vi "MCCETC01_Main.vi"(7 "stop_external":refnum<vi>) -> ()   [LabVIEW 2019]
uses:
  MCCETC_Global.vi
panel:
  out "T7":dbl format="%.2f"
  in  "Logging":bool=TRUE
  out "status_log":bool caption="Status"
  out "T6":dbl format="%.2f"
  out "T5":dbl format="%.2f"
  out "T4":dbl format="%.2f"
  out "T3":dbl format="%.2f"
  out "T2":dbl format="%.2f"
  in  "Tab Control":enum32{"Top Coil", "Bottom Coil"}(tab)
  out "T0 Chart":waveform(dbl)[](graph)
  out "T1 Chart":waveform(dbl)[](graph)
  out "T2 Chart":waveform(dbl)[](graph)
  out "T3 Chart":waveform(dbl)[](graph)
  out "T4 Chart":waveform(dbl)[](graph)
  out "T5 Chart":waveform(dbl)[](graph)
  out "T6 Chart":waveform(dbl)[](graph)
  out "T7 Chart":waveform(dbl)[](graph)
  in  "Readout Interval":i32=5 caption="sec"
  in  "units":i32(ring)=2 items=["degC", "degF", "kelvin", "raw"]
  out "T1":dbl format="%.2f"
  out "T0":dbl format="%.2f"
  out "Readout Status":bool
  out "Last Measured":timestamp format="%<%Y-%m-%d %H:%M:%S>T"
  in  "stop":bool
  # "MCC E-TC #01:  Target Magnet Coil"
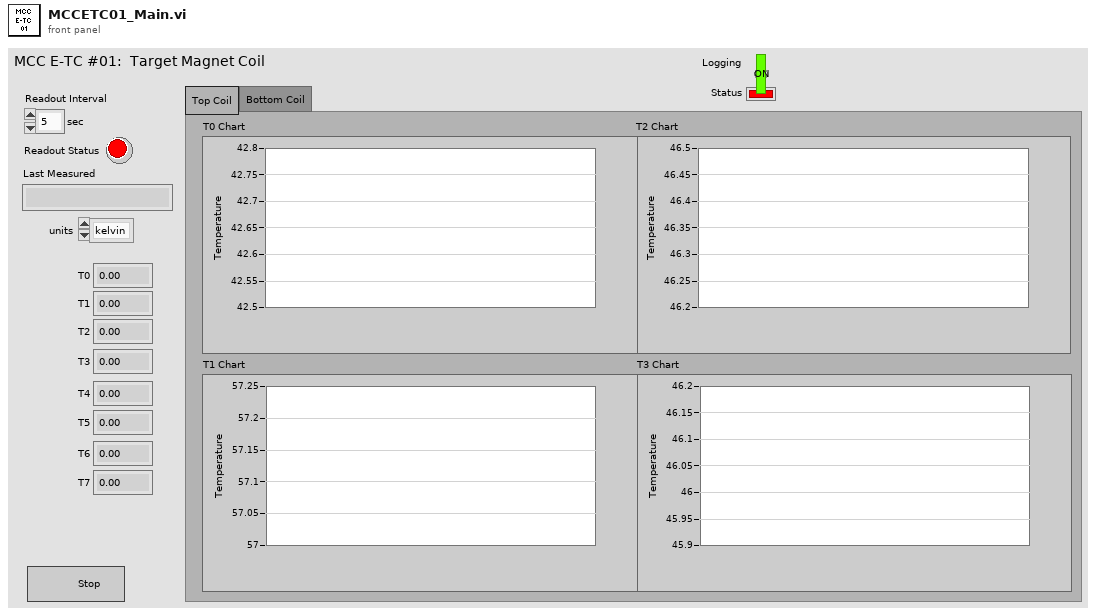
[diagram p1: front panel]
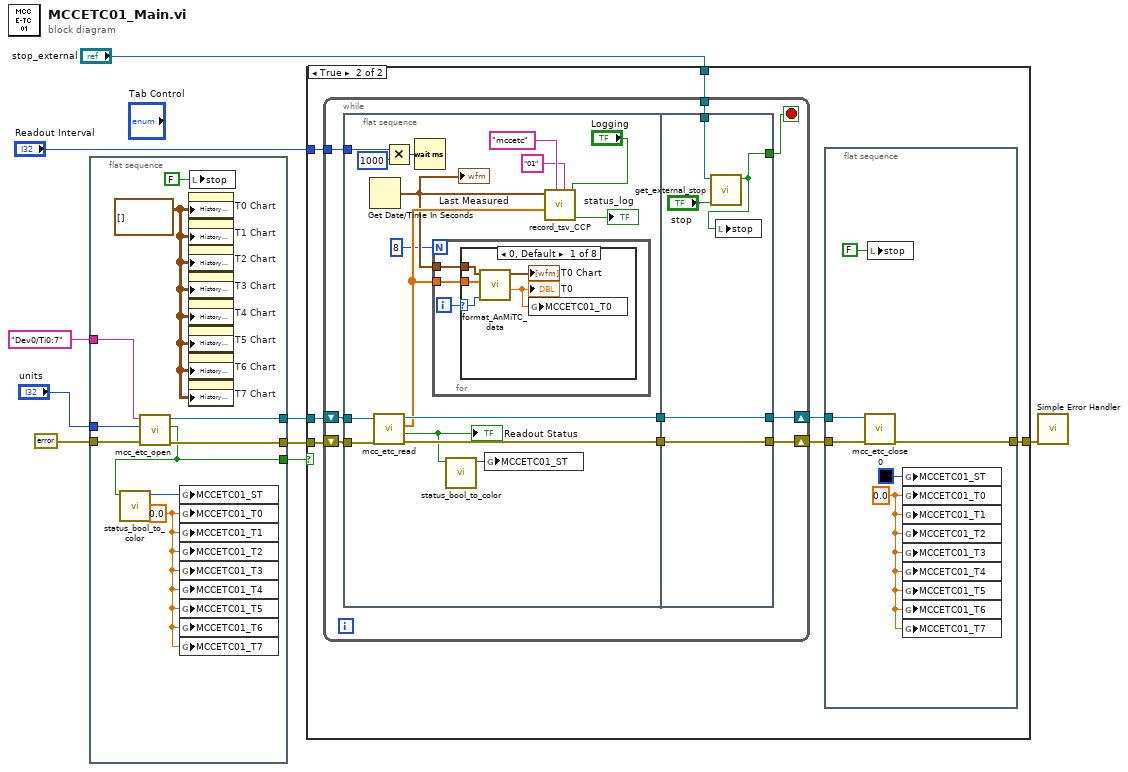
[diagram p0: block diagram]
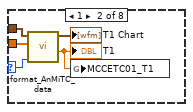
[diagram p3: hidden frame]
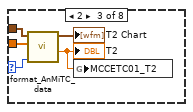
[diagram p4: hidden frame]
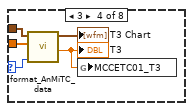
[diagram p5: hidden frame]
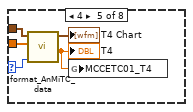
[diagram p6: hidden frame]
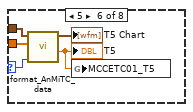
[diagram p7: hidden frame]
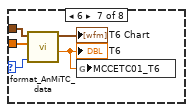
[diagram p8: hidden frame]
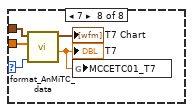
[diagram p9: hidden frame]
diagram:
  n1 = flat-sequence {
    tunnel: [w19] -> w9
    tunnel: errorcluster {"status"=FALSE, "code"=0, "source"=""} ("error in") -> [w18]
    tunnel: [w17] -> w7
    tunnel: "Dev0/Ti0:7" ("Device/Channel Name") -> [w16]
    tunnel: "units" -> [w15]
    tunnel: [w10] -> w2
    frame #0 {
      w12 = 0.0 ("MCCETC01_T0")
      w13 = waveform(dbl)[][] [] ("History Data")
      n2 = call "mcc_etc_open.vi"("error in"=w18, "units"=w15, "name"=w16) -> ("error out"=w17:errorcluster, "status"=w10:bool, "task out"=w19:refnum<k24>)  [unwired: 6 in]
      n3 = call "status_bool_to_color.vi"("status_bool_1"=w10) -> ("status_color"=w11:u32)  [unwired: 10 in]
      n4 = global write "MCCETC_Global.vi" "MCCETC01_ST"(w11) -> ()
      n5 = global write "MCCETC_Global.vi" "MCCETC01_T0"(w12) -> ()
      n6 = global write "MCCETC_Global.vi" "MCCETC01_T1"(w12) -> ()
      n7 = global write "MCCETC_Global.vi" "MCCETC01_T2"(w12) -> ()
      n8 = global write "MCCETC_Global.vi" "MCCETC01_T3"(w12) -> ()
      n9 = global write "MCCETC_Global.vi" "MCCETC01_T4"(w12) -> ()
      n10 = global write "MCCETC_Global.vi" "MCCETC01_T5"(w12) -> ()
      n11 = global write "MCCETC_Global.vi" "MCCETC01_T6"(w12) -> ()
      n12 = global write "MCCETC_Global.vi" "MCCETC01_T7"(w12) -> ()
      n13 = property on="T0 Chart" class="WFChart (strict)"("History Data"=w13) -> ()  [unwired: 2 in, 2 out]
      n14 = property on="T1 Chart" class="WFChart (strict)"("History Data"=w13) -> ()  [unwired: 2 in, 2 out]
      n15 = property on="T2 Chart" class="WFChart (strict)"("History Data"=w13) -> ()  [unwired: 2 in, 2 out]
      n16 = property on="T3 Chart" class="WFChart (strict)"("History Data"=w13) -> ()  [unwired: 2 in, 2 out]
      n17 = property on="T4 Chart" class="WFChart (strict)"("History Data"=w13) -> ()  [unwired: 2 in, 2 out]
      n18 = property on="T5 Chart" class="WFChart (strict)"("History Data"=w13) -> ()  [unwired: 2 in, 2 out]
      n19 = property on="T6 Chart" class="WFChart (strict)"("History Data"=w13) -> ()  [unwired: 2 in, 2 out]
      n20 = property on="T7 Chart" class="WFChart (strict)"("History Data"=w13) -> ()  [unwired: 2 in, 2 out]
      n21 = local write "stop"(FALSE ("Stop")) -> ()
    }
  }
  n22 = case shown="True" w2 {
    tunnel: w9 -> [_ w27]
    tunnel: w7 -> [w20 w26]
    tunnel: "Readout Interval" -> [_ w23]
    tunnel: [w20 w22] -> w3
    tunnel: "stop_external" -> [_ w21]
    frame False {
    }
    frame True {
      n23 = while {
        shift-right: [w40] -> w24
        shift-left: w26 -> [w41]
        shift-right: [w39] -> w25
        shift-left: w27 -> [w42]
        tunnel: w23 -> [w38]
        tunnel: w21 -> [w34]
        stop <- w35 stop-if-true
        n24 = flat-sequence {
          tunnel: w42 -> [w58]
          tunnel: w41 -> [w57]
          tunnel: w38 -> [w54]
          tunnel: [w56] -> w37
          tunnel: [w55] -> w36
          tunnel: [w105] -> w39
          tunnel: [w106] -> w40
          tunnel: w37 -> [w106]
          tunnel: w36 -> [w105]
          tunnel: [w103] -> w35
          tunnel: w34 -> [w102]
          frame #0 {
            n25 = Get Date/Time In Seconds() -> (seconds since 1Jan1904=w45:timestamp)
            "Last Measured" <- w45
            n26 = call "mcc_etc_read.vi"("error in"=w57, "task in"=w58) -> ("error out"=w56:errorcluster, "status"=w47:bool, "temperature_array"=w46:dbl[], "task out"=w55:refnum<k24>)  [unwired: 6 in]
            "Readout Status" <- w47
            n27 = Multiply(x=w54, y=1000) -> (x*y=w53:i32)
            n28 = Wait (ms)(milliseconds to wait=w53) -> ()  [unwired: 1 out]
            n29 = for {
              N: 8 -> [_]
              tunnel: w46 -> [w60]
              tunnel: w45 -> [w59]
              i -> [w61]
              n30 = case shown="0, Default" w61 {
                selector: w61 -> [w65 w69 w74 w79 w84 w89 w94 w99]
                tunnel: w60 -> [w66 w71 w76 w81 w86 w91 w96 w101]
                tunnel: w59 -> [w64 w70 w75 w80 w85 w90 w95 w100]
                frame 0, Default {
                  n31 = call "format_AnMiTC_data.vi"("index"=w65, "value_array"=w66, "time"=w64) -> ("value"=w62:dbl, "waveform_array"=→"T0 Chart":waveform(dbl)[])  [unwired: 7 in]
                  "T0" <- w62
                  n32 = global write "MCCETC_Global.vi" "MCCETC01_T0"(w62) -> ()
                }
                frame 1 {
                  n33 = call "format_AnMiTC_data.vi"("index"=w69, "value_array"=w71, "time"=w70) -> ("value"=w67:dbl, "waveform_array"=→"T1 Chart":waveform(dbl)[])  [unwired: 7 in]
                  "T1" <- w67
                  n34 = global write "MCCETC_Global.vi" "MCCETC01_T1"(w67) -> ()
                }
                frame 2 {
                  n35 = call "format_AnMiTC_data.vi"("index"=w74, "value_array"=w76, "time"=w75) -> ("value"=w72:dbl, "waveform_array"=→"T2 Chart":waveform(dbl)[])  [unwired: 7 in]
                  "T2" <- w72
                  n36 = global write "MCCETC_Global.vi" "MCCETC01_T2"(w72) -> ()
                }
                frame 3 {
                  n37 = call "format_AnMiTC_data.vi"("index"=w79, "value_array"=w81, "time"=w80) -> ("value"=w77:dbl, "waveform_array"=→"T3 Chart":waveform(dbl)[])  [unwired: 7 in]
                  "T3" <- w77
                  n38 = global write "MCCETC_Global.vi" "MCCETC01_T3"(w77) -> ()
                }
                frame 4 {
                  n39 = call "format_AnMiTC_data.vi"("index"=w84, "value_array"=w86, "time"=w85) -> ("value"=w82:dbl, "waveform_array"=→"T4 Chart":waveform(dbl)[])  [unwired: 7 in]
                  "T4" <- w82
                  n40 = global write "MCCETC_Global.vi" "MCCETC01_T4"(w82) -> ()
                }
                frame 5 {
                  n41 = call "format_AnMiTC_data.vi"("index"=w89, "value_array"=w91, "time"=w90) -> ("value"=w87:dbl, "waveform_array"=→"T5 Chart":waveform(dbl)[])  [unwired: 7 in]
                  "T5" <- w87
                  n42 = global write "MCCETC_Global.vi" "MCCETC01_T5"(w87) -> ()
                }
                frame 6 {
                  n43 = call "format_AnMiTC_data.vi"("index"=w94, "value_array"=w96, "time"=w95) -> ("value"=w92:dbl, "waveform_array"=→"T6 Chart":waveform(dbl)[])  [unwired: 7 in]
                  "T6" <- w92
                  n44 = global write "MCCETC_Global.vi" "MCCETC01_T6"(w92) -> ()
                }
                frame 7 {
                  n45 = call "format_AnMiTC_data.vi"("index"=w99, "value_array"=w101, "time"=w100) -> ("value"=w97:dbl, "waveform_array"=→"T7 Chart":waveform(dbl)[])  [unwired: 7 in]
                  "T7" <- w97
                  n46 = global write "MCCETC_Global.vi" "MCCETC01_T7"(w97) -> ()
                }
              }
            }
            n47 = call "status_bool_to_color.vi"("status_bool_1"=w47) -> ("status_color"=w44:u32)  [unwired: 10 in]
            n48 = global write "MCCETC_Global.vi" "MCCETC01_ST"(w44) -> ()
            n49 = call "record_tsv_CCP.vi"("logging_on"="Logging", "file_name"="01", "folder_name"="mccetc", "value_array"=w46, "time"=w45) -> ("status"=→"status_log":bool)  [unwired: 5 in, 1 out]
          }
          frame #1 {
            n50 = call "get_external_stop.vi"("stop_internal"="stop", "ref_stop_external"=w102) -> ("stop_output"=w103:bool)  [unwired: 9 in]
            n51 = local write "stop"(w103) -> ()
          }
        }
      }
      n52 = flat-sequence {
        tunnel: w25 -> [w33]
        tunnel: w24 -> [w32]
        tunnel: [w31] -> w22
        frame #0 {
          w29 = 0.0 ("MCCETC01_T0")
          n53 = call "mcc_etc_close.vi"("error in"=w32, "task in"=w33) -> ("error out"=w31:errorcluster)  [unwired: 8 in, 1 out]
          n54 = local write "stop"(FALSE ("Stop")) -> ()
          n55 = global write "MCCETC_Global.vi" "MCCETC01_ST"(u32 0 ("MCCETC01_ST")) -> ()
          n56 = global write "MCCETC_Global.vi" "MCCETC01_T0"(w29) -> ()
          n57 = global write "MCCETC_Global.vi" "MCCETC01_T1"(w29) -> ()
          n58 = global write "MCCETC_Global.vi" "MCCETC01_T2"(w29) -> ()
          n59 = global write "MCCETC_Global.vi" "MCCETC01_T3"(w29) -> ()
          n60 = global write "MCCETC_Global.vi" "MCCETC01_T4"(w29) -> ()
          n61 = global write "MCCETC_Global.vi" "MCCETC01_T5"(w29) -> ()
          n62 = global write "MCCETC_Global.vi" "MCCETC01_T6"(w29) -> ()
          n63 = global write "MCCETC_Global.vi" "MCCETC01_T7"(w29) -> ()
        }
      }
    }
  }
  n64 = call <vilib>:"Simple Error Handler.vi"("error in (no error)"=w3) -> ()  [unwired: 4 in, 5 out]
